vi "Wait on Notifier.vi"(8 "Error In":errorcluster, 9 "timeout in ms (-1)":i32, 11 "notifier in":refnum<notifier>) -> (0 "Error Out":errorcluster, 3 "notifier out":refnum<notifier>)   [LabVIEW 2019, in "Error Notifier.lvlib"]
uses:
  Error Notifier.lvlib
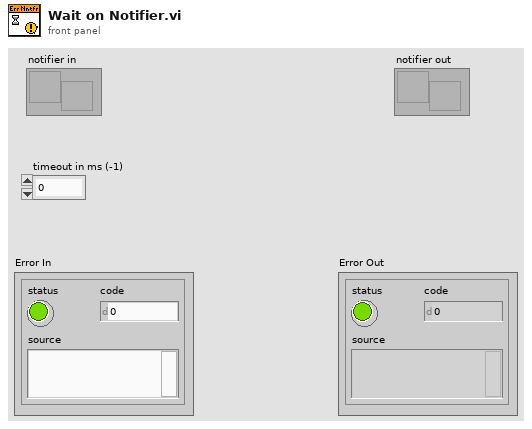
[diagram p1: front panel]
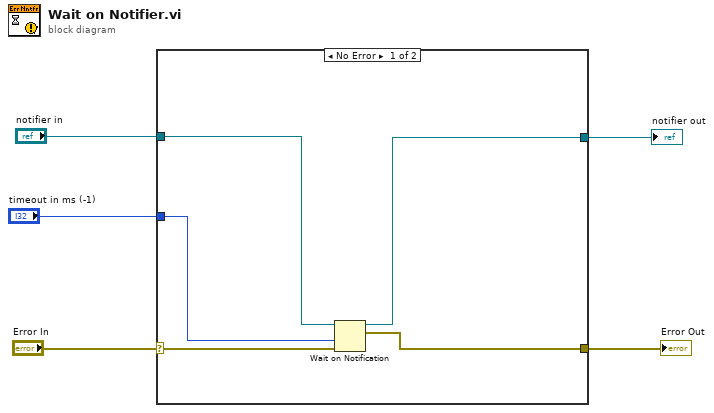
[diagram p0: block diagram]
diagram:
  n1 = case shown="No Error" "Error In" {
    selector: "Error In" -> [w10 w12]
    tunnel: [w7 w12] -> w4
    tunnel: "notifier in" -> [w9 w11]
    tunnel: [w8 w11] -> w2
    tunnel: "timeout in ms (-1)" -> [w6 _]
    frame No Error {
      n2 = Wait on Notification(notifier=w9, timeout in ms (-1)=w6, error in (no error)=w10) -> (notifier out=w8:refnum<notifier>, notification=w7:errorcluster)  [unwired: 1 in, 2 out]
    }
    frame Error {
    }
  }
  "Error Out" <- w4
  "notifier out" <- w2
